vi "1DTurnMainTester.vi"() -> ()   [LabVIEW 2017]
uses:
  <vilib>/Rock Robotics/WPI/SafetyOutput/WPI_SafetyOutputConfigMenu.ctl
  <vilib>/Rock Robotics/SystemInterfaces/DIO/FPGA_DIOPWMChannel.ctl
  <vilib>/Rock Robotics/SystemInterfaces/DIO/FPGA_DIOChannel.ctl
  <extravilib>/ChannelInstances/Lossy Stream-c(dbl,dbl,dbl,dbl,dbl,dbl)/Write With Abort.vi
  <extravilib>/ChannelInstances/Lossy Stream-c(dbl,dbl,dbl,dbl,dbl,dbl)/Read With Abort.vi
  <extravilib>/ChannelInstances/Lossy Stream-c(dbl,dbl,dbl,dbl,dbl,dbl)/Endpoint.vi
  <extravilib>/ChannelInstances/Lossy Stream-c(dbl,dbl,dbl,dbl,dbl,dbl)/EndpointRead.vi
  <vilib>/Rock Robotics/WPI/RobotDrive/WPI_RobotDriveOpen4MotorWithSPARK.vi
  <vilib>/Rock Robotics/WPI/RobotDrive/WPI_RobotDriveOpen2MotorWithSPARK.vi
  <vilib>/Rock Robotics/WPI/Counter/WPI_CounterDigitalInputToDigitalSource.vi
  <extravilib>/ChannelInstances/Lossy Stream-c(dbl,dbl,dbl,dbl,dbl,dbl)/Instantiate.vi
  <extravilib>/ChannelInstances/Lossy Stream-c(dbl,dbl,dbl,dbl,dbl,dbl)/)Channel.vi
  <resource>/ChannelSupport/_ChannelSupport/WaitIfNeeded.vi
  <vilib>/Rock Robotics/WPI/ThirdParty/Sensors/navX/_Processing Loop/FRIC_navX_Internal_SPI_ProcessingLoop.vi
  <extravilib>/ChannelInstances/Lossy Stream-c(dbl,dbl,dbl,dbl,dbl,dbl).lvlib
panel:
  out "Trackwidth":dbl(graph)
  in  "AutoTurnSpeed":dbl=0.55
  in  "ThingToDo":enum16{"TestTurning", "FindTrackwidth"}(ring)
  out "Encoder Position":cluster{"Distance":dbl, "CurrentAngle":dbl}(graph)={"Distance"=0.0, "CurrentAngle"=7.280000000000058}
  in  "Gains":T1={"Gains"={"FFV"=0.0059, "FFA"=0.0019, "Vel PID"={"P"=0.01, "I"=0.0, "D"=0.0}}, "Pos PID"={"P"=0.02, "I"=0.0, "D"=0.0}, "MinVoltage"=0.0, "Effective Trackwidth"=30.0} {"Pos PID"."D" format="%.3f"; "Pos PID"."I" format="%.3f"; "Pos PID"."P" format="%.3f"}
  in  "A? or B":bool=TRUE
  in  "TargetB":dbl=500.0
  out "Voltage difference":dbl(graph)=1.0
  out "Power":dbl(graph)
  out "Done?":bool
  out "Vel":cluster{"Output":dbl, "dx/dt":dbl}(graph)
  out "Angle":cluster{"Distance":dbl, "CurrentAngle":dbl}(graph)={"Distance"=0.0, "CurrentAngle"=6.750000000000796}
  in  "TargetA":dbl
  in  "MaxVel":dbl=130.0
  in  "MaxAccel":dbl=120.0
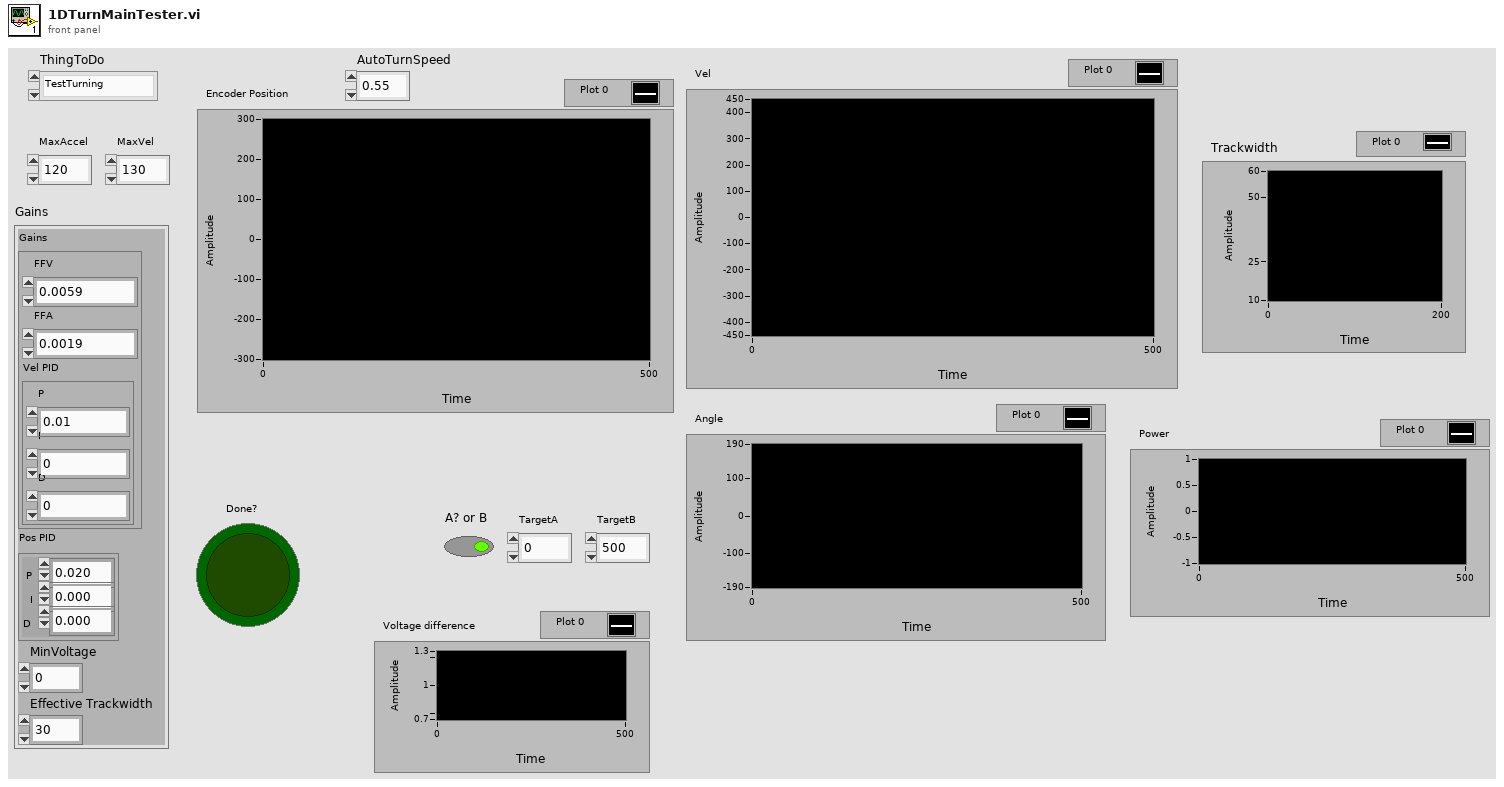
[diagram p1: front panel]
types:
  T1 = cluster{"Gains":cluster{"FFV":dbl, "FFA":dbl, "Vel PID":cluster{"P":dbl, "I":dbl, "D":dbl}}, "Pos PID":cluster{"P":dbl, "I":dbl, "D":dbl}, "MinVoltage":dbl, "Effective Trackwidth":dbl}
  T2 = typedef "FPGA_DIOChannel.ctl" = enum8{"DIO 0", "DIO 1", "DIO 2", "DIO 3", "DIO 4", "DIO 5", "DIO 6", "DIO 7", "DIO 8", "DIO 9", "DIO MXP 0", "DIO MXP 1", "DIO MXP 2", "DIO MXP 3", "DIO MXP 4", "DIO MXP 5", "DIO MXP 6", "DIO MXP 7", "DIO MXP 8", "DIO MXP 9", "DIO MXP 10", "DIO MXP 11", "DIO MXP 12", "DIO MXP 13", "DIO MXP 14", "DIO MXP 15", "SPI Port CS1", "SPI Port CS2", "SPI Port CS3", "SPI Port MISO", "SPI Port MOSI", "Invalid"}
  T3 = typedef "FPGA_DIOPWMChannel.ctl" = enum8{"PWM 0", "PWM 1", "PWM 2", "PWM 3", "PWM 4", "PWM 5", "PWM 6", "PWM 7", "PWM 8", "PWM 9", "PWM MXP 0", "PWM MXP 1", "PWM MXP 2", "PWM MXP 3", "PWM MXP 4", "PWM MXP 5", "PWM MXP 6", "PWM MXP 7", "PWM MXP 8", "PWM MXP 9", "Invalid"}
  T4 = typedef "WPI_SafetyOutputConfigMenu.ctl" = enum16{"Enable", "Disable"}
  T5 = typedef "WPI_DigitalInputDevRef.ctl" = cluster{"DevStatus":errorcluster, "DIO Channel":T2}
  T6 = typedef "FPGA_CounterEncoderSourceConvertionLVSourceType.ctl" = cluster{"DevStatus":errorcluster, "AnalogTriggerMode?":bool, "DigitalMode":cluster{"DIO Channel":T7}, "AnalogTriggerMode":cluster{"AnalogTriggerIndex":T8, "OutputType":T9}}
  T7 = typedef "FPGA_DIODigitalSourceChannel.ctl" = enum8{"DIO 0", "DIO 1", "DIO 2", "DIO 3", "DIO 4", "DIO 5", "DIO 6", "DIO 7", "DIO 8", "DIO 9", "DIO MXP 0", "DIO MXP 1", "DIO MXP 2", "DIO MXP 3", "DIO MXP 4", "DIO MXP 5", "DIO MXP 6", "DIO MXP 7", "DIO MXP 8", "DIO MXP 9", "DIO MXP 10", "DIO MXP 11", "DIO MXP 12", "DIO MXP 13", "DIO MXP 14", "DIO MXP 15", "Disabled"}
  T8 = typedef "FPGA_AnalogTriggerIndex.ctl" = enum8{"Trig 0", "Trig 1", "Trig 2", "Trig 3", "Trig 4", "Trig 5", "Trig 6", "Trig 7", "Invalid"}
  T9 = typedef "FPGA_AnalogTriggerOutType.ctl" = enum16{"InWindow", "TriggerState", "Rising", "Falling"}
  T10 = typedef "WPI_EncoderDevRef.ctl" = cluster{"DevStatus":errorcluster, "EncoderIndex":T11, "CounterIndex":T12, "DistancePerCount":dbl, "Decoding Type":T13}
  T11 = typedef "FPGA_EncoderIdx.ctl" = enum8{"Enc 0", "Enc 1", "Enc 2", "Enc 3", "Enc 4", "Enc 5", "Enc 6", "Enc 7", "Invalid"}
  T12 = typedef "FPGA_CounterCtrSystemIndex.ctl" = enum8{"Ctr 0", "Ctr 1", "Ctr 2", "Ctr 3", "Ctr 4", "Ctr 5", "Ctr 6", "Ctr 7", "Invalid"}
  T13 = typedef "WPI_EncoderType.ctl" = enum16{"1x", "2x", "4x"}
  T14 = typedef "WPI_RobotDriveDevRef.ctl" = cluster{"DevStatus":errorcluster, "Motors[]":T15[], "Square Inputs":bool, "Max Output":dbl}
  T15 = typedef "WPI_MotorControlDeviceRef.ctl" = cluster{"DeviceStatus":errorcluster, "Type":T16, "PWM":cluster{"PWM Channel":T3, "DeadBand":T17}, "CAN":cluster{"Device Number":u8, "SetOutput VI Ref":variant, "GetOutput VI Ref":variant, "Enable VI Ref":variant, "Disable VI Ref":variant, "Data":variant}, "Invert":bool, "DIO PWM":cluster{"PWM \"Enable\" Channel":T3, "DIOChannel":T2, "PWM Rate":dbl}}
  T16 = typedef "WPI_MotorControlType.ctl" = enum16{"PWM", "CAN", "DIO PWM"}
  T17 = typedef "WPI_PWMDeadband.ctl" = cluster{"Name":string, "maxPositivePwm":i32, "minPositivePwm":i32, "centerPwm":i32, "maxNegativePwm":i32, "minNegativePwm":i32, "angularRange":u16}
  T18 = cluster{"Yaw":dbl, "Roll":dbl, "Pitch":dbl, "Heading":dbl, "Fused Heading":dbl}
  T19 = cluster{dbl, "dx/dt":dbl, "Distance":dbl, "dx/dt":dbl, "Distance":dbl, "dx/dt":dbl}
  T20 = typedef "Lossy Stream-c(dbl,dbl,dbl,dbl,dbl,dbl).lvlib/)Channel.ctl" = refnum<queue>
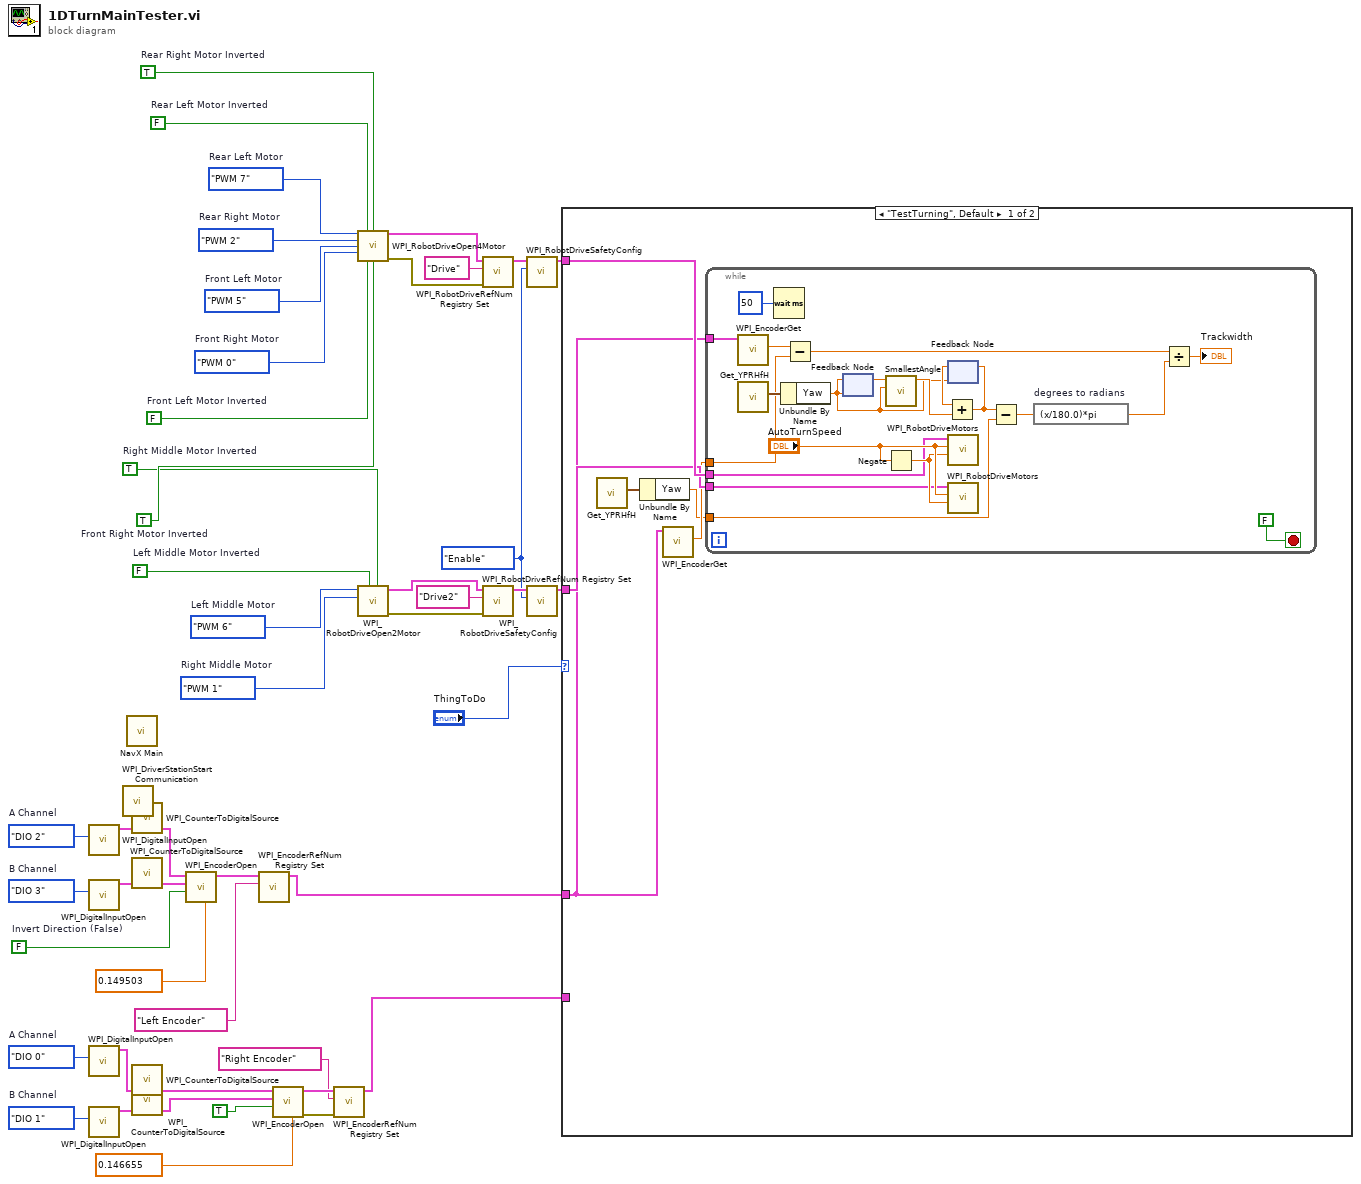
[diagram p0: block diagram]
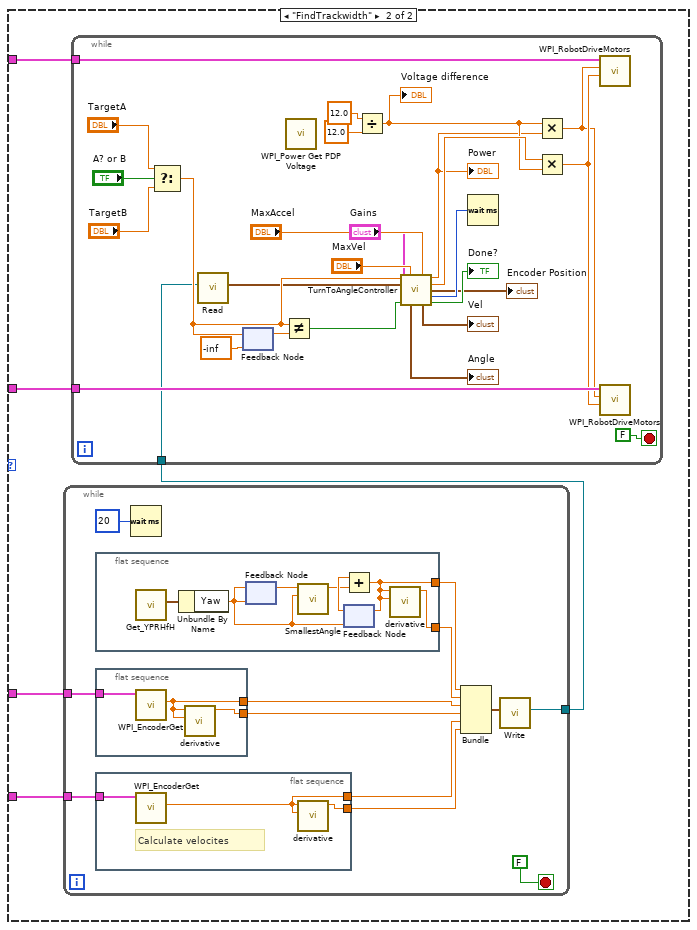
[diagram p2: hidden frame]
diagram:
  w7 = FPGA_DIOChannel."DIO 1"  # B Channel
  w10 = FPGA_DIOChannel."DIO 0"  # A Channel
  w23 = FALSE  # Invert Direction (False)
  w16 = FPGA_DIOChannel."DIO 3"  # B Channel
  w17 = FPGA_DIOChannel."DIO 2"  # A Channel
  w32 = TRUE  # Right Middle Motor Inverted
  w33 = FALSE  # Left Middle Motor Inverted
  w27 = FPGA_DIOPWMChannel."PWM 1"  # Right Middle Motor
  w36 = FPGA_DIOPWMChannel."PWM 6"  # Left Middle Motor
  w37 = TRUE  # Front Right Motor Inverted
  w38 = FALSE  # Front Left Motor Inverted
  w39 = TRUE  # Rear Right Motor Inverted
  w40 = FALSE  # Rear Left Motor Inverted
  w41 = FPGA_DIOPWMChannel."PWM 0"  # Front Right Motor
  w42 = FPGA_DIOPWMChannel."PWM 5"  # Front Left Motor
  w43 = FPGA_DIOPWMChannel."PWM 2"  # Rear Right Motor
  w44 = FPGA_DIOPWMChannel."PWM 7"  # Rear Left Motor
  w28 = WPI_SafetyOutputConfigMenu."Enable" ("mode")
  n1 = call <vilib>:"WPI_DigitalInputOpen.vi"("DIO Channel"=w17) -> ("DigitalInputDevRef"=w20:T5)  [unwired: 1 in, 9 out]
  n2 = call <vilib>:"WPI_DigitalInputOpen.vi"("DIO Channel"=w16) -> ("DigitalInputDevRef"=w19:T5)  [unwired: 1 in, 9 out]
  n3 = call <vilib>:"WPI_DigitalInputOpen.vi"("DIO Channel"=w10) -> ("DigitalInputDevRef"=w11:T5)  [unwired: 1 in, 9 out]
  n4 = call <vilib>:"WPI_DigitalInputOpen.vi"("DIO Channel"=w7) -> ("DigitalInputDevRef"=w8:T5)  [unwired: 1 in, 9 out]
  n5 = call <vilib>:"WPI_DriverStationStart Communication.vi"() -> ()  [unwired: 12 in]
  n6 = call-poly <vilib>:"NavX Main.vi"() -> ()  [unwired: 12 in]
  n7 = call-poly <vilib>:"WPI_CounterToDigitalSource.vi"("DigitalInputDevRef"=w20) -> ("Digital Source"=w21:T6)  [unwired: 6 out]
  n8 = call-poly <vilib>:"WPI_CounterToDigitalSource.vi"("DigitalInputDevRef"=w19) -> ("Digital Source"=w18:T6)  [unwired: 6 out]
  n9 = call-poly <vilib>:"WPI_CounterToDigitalSource.vi"("DigitalInputDevRef"=w11) -> ("Digital Source"=w12:T6)  [unwired: 6 out]
  n10 = call-poly <vilib>:"WPI_CounterToDigitalSource.vi"("DigitalInputDevRef"=w8) -> ("Digital Source"=w9:T6)  [unwired: 6 out]
  n11 = call <vilib>:"WPI_EncoderOpen.vi"("DistancePerCount"=0.149503, "Invert Direction (False)"=w23, "BSource"=w18, "ASource"=w21) -> ("EncoderDevRef"=w22:T10)  [unwired: 4 in, 3 out]
  n12 = call <vilib>:"WPI_EncoderRefNum Registry Set.vi"("refnum name"="Left Encoder", "EncoderDevRef"=w22) -> ("EncoderDevRef"=w3:T10)  [unwired: 8 in, 1 out]
  n13 = call <vilib>:"WPI_EncoderOpen.vi"("DistancePerCount"=0.146655, "Invert Direction (False)"=TRUE, "BSource"=w9, "ASource"=w12) -> ("error out"=w14:errorcluster, "EncoderDevRef"=w13:T10)  [unwired: 4 in, 2 out]
  n14 = call <vilib>:"WPI_EncoderRefNum Registry Set.vi"("error in (no error)"=w14, "refnum name"="Right Encoder", "EncoderDevRef"=w13) -> ("EncoderDevRef"=w2:T10)  [unwired: 7 in, 1 out]
  n15 = call-poly <vilib>:"WPI_RobotDriveOpen4Motor.vi"("Rear Left Motor"=w44, "Rear Left Motor Inverted"=w40, "Rear Right Motor Inverted"=w39, "Rear Right Motor"=w43, "Front Left Motor"=w42, "Front Right Motor"=w41, "Front Left Motor Inverted"=w38, "Front Right Motor Inverted"=w37) -> ("RobotDriveDevRef"=w47:T14, "error out"=w45:errorcluster)  [unwired: 6 in]
  n16 = call-poly <vilib>:"WPI_RobotDriveOpen2Motor.vi"("Right Motor Inverted"=w32, "Left Motor Inverted"=w33, "Right Motor"=w27, "Left Motor"=w36) -> ("error out"=w31:errorcluster, "RobotDriveDevRef"=w35:T14)  [unwired: 6 in]
  n17 = call <vilib>:"WPI_RobotDriveRefNum Registry Set.vi"("error in (no error)"=w45, "refnum name"="Drive", "RobotDriveDevRef"=w47) -> ("RobotDriveDevRef"=w30:T14)  [unwired: 1 in, 7 out]
  n18 = call <vilib>:"WPI_RobotDriveRefNum Registry Set.vi"("error in (no error)"=w31, "refnum name"="Drive2", "RobotDriveDevRef"=w35) -> ("RobotDriveDevRef"=w29:T14)  [unwired: 7 in, 1 out]
  n19 = call <vilib>:"WPI_RobotDriveSafetyConfig.vi"("mode"=w28, "RobotDriveDevRef"=w30) -> ("RobotDriveDevRef"=w25:T14)  [unwired: 8 in, 1 out]
  n20 = call <vilib>:"WPI_RobotDriveSafetyConfig.vi"("mode"=w28, "RobotDriveDevRef"=w29) -> ("RobotDriveDevRef"=w26:T14)  [unwired: 8 in, 1 out]
  n21 = case shown="\"TestTurning\", Default" "ThingToDo" {
    tunnel: w26 -> [w52 w78]
    tunnel: w25 -> [w53 w77]
    tunnel: w3 -> [w51 w76]
    tunnel: w2 -> [_ w75]
    frame "TestTurning", Default {
      n22 = call <vilib>:"Get_YPRHfH.vi"() -> ("YRPHfH"=w49:T18)  [unwired: 11 in]
      n23 = Unbundle By Name(w49) -> ("Yaw"=w48:dbl)
      n24 = call <vilib>:"WPI_EncoderGet.vi"("EncoderDevRef"=w51) -> ("Distance"=w50:dbl)  [unwired: 5 in, 5 out]
      n25 = while {
        tunnel: w53 -> [w69]
        tunnel: w52 -> [w68]
        tunnel: w51 -> [w62]
        tunnel: w50 -> [w60]
        tunnel: w48 -> [w58]
        stop <- FALSE stop-if-true
        n26 = call <vilib>:"WPI_EncoderGet.vi"("EncoderDevRef"=w62) -> ("Distance"=w61:dbl)  [unwired: 5 in, 5 out]
        n27 = call <vilib>:"Get_YPRHfH.vi"() -> ("YRPHfH"=w67:T18)  [unwired: 11 in]
        n28 = Wait (ms)(milliseconds to wait=u32 50) -> ()  [unwired: 1 out]
        n29 = Unbundle By Name(w67) -> ("Yaw"=w63:dbl)
        n30 = Subtract(x=w61, y=w60) -> (x-y=w56:dbl)
        n31 = feedback #1(w63) -> (w64:dbl)
        n32 = feedback-in #1(w63) -> ()
        n33 = call "SmallestAngle.vi"("Angle B"=w63, "Angle A"=w64) -> ("Smallest A to B"=w65:dbl)  [unwired: 9 in]
        n34 = Negate(x="AutoTurnSpeed") -> (-x=w72:dbl)
        n35 = feedback #2(w63) -> (w66:dbl)
        n36 = Add(x=w66, y=w65) -> (x+y=w59:dbl)
        n37 = feedback-in #2(w59) -> ()
        n38 = call <vilib>:"WPI_RobotDriveMotors.vi"("RightSpeed"=w72, "LeftSpeed"="AutoTurnSpeed", "RobotDriveDevRef"=w69) -> ()  [unwired: 1 in, 8 out]
        n39 = call <vilib>:"WPI_RobotDriveMotors.vi"("RightSpeed"=w72, "LeftSpeed"="AutoTurnSpeed", "RobotDriveDevRef"=w68) -> ()  [unwired: 1 in, 8 out]
        n40 = Subtract(x=w59, y=w58) -> (x-y=w57:dbl)
        n41 = expression code="(x/180.0)*pi" "degrees to radians"(w57) -> (w55:dbl)
        n42 = Divide(x=w56, y=w55) -> (x/y=→"Trackwidth":dbl)
      }
    }
    frame "FindTrackwidth" {
      n43 = while {
        tunnel: w76 -> [w86]
        tunnel: w75 -> [w85]
        tunnel: [w79] -> w74
        stop <- FALSE stop-if-true
        n44 = flat-sequence {
          tunnel: [w102] -> w87
          tunnel: [w98] -> w88
          frame #0 {
            n45 = call <vilib>:"Get_YPRHfH.vi"() -> ("YRPHfH"=w103:T18)  [unwired: 11 in]
            n46 = Unbundle By Name(w103) -> ("Yaw"=w97:dbl)
            n47 = feedback #3(w97) -> (w99:dbl)
            n48 = feedback-in #3(w97) -> ()
            n49 = call "SmallestAngle.vi"("Angle B"=w97, "Angle A"=w99) -> ("Smallest A to B"=w100:dbl)  [unwired: 9 in]
            n50 = feedback #4(w97) -> (w101:dbl)
            n51 = Add(x=w101, y=w100) -> (x+y=w98:dbl)
            n52 = feedback-in #4(w98) -> ()
            n53 = call "derivative.vi"("Starting value"=w98, "x"=w98) -> ("dx/dt"=w102:dbl)  [unwired: 9 in]
          }
        }
        n54 = flat-sequence {
          tunnel: [w93] -> w83
          tunnel: [w92] -> w84
          tunnel: w86 -> [w91]
          frame #0 {
            n55 = call <vilib>:"WPI_EncoderGet.vi"("EncoderDevRef"=w91) -> ("Distance"=w92:dbl)  [unwired: 5 in, 5 out]
            n56 = call "derivative.vi"("Starting value"=w92, "x"=w92) -> ("dx/dt"=w93:dbl)  [unwired: 9 in]
          }
        }
        n57 = flat-sequence {
          tunnel: [w95] -> w81
          tunnel: [w94] -> w82
          tunnel: w85 -> [w96]
          frame #0 {
            # "Calculate velocites"
            n58 = call <vilib>:"WPI_EncoderGet.vi"("EncoderDevRef"=w96) -> ("Distance"=w94:dbl)  [unwired: 5 in, 5 out]
            n59 = call "derivative.vi"("Starting value"=w94, "x"=w94) -> ("dx/dt"=w95:dbl)  [unwired: 9 in]
          }
        }
        n60 = Wait (ms)(milliseconds to wait=u32 20) -> ()  [unwired: 1 out]
        n61 = Bundle(w88, "dx/dt"=w87, "Distance"=w84, "dx/dt"=w83, "Distance"=w82, "dx/dt"=w81) -> (w80:T19)  [unwired: 1 in]
        n62 = call <extravilib>:"Write.vi"("element"=w80) -> ("channel"=w79:T20)  [unwired: 8 in, 2 out]
      }
      n63 = while {
        tunnel: w78 -> [w121]
        tunnel: w77 -> [w120]
        tunnel: w74 -> [w108]
        stop <- FALSE stop-if-true
        n64 = Select(t="TargetA", s="A? or B", f="TargetB") -> (s? t:f=w109:dbl)
        n65 = call <extravilib>:"Read.vi"("channel"=w108) -> ("element"=w107:T19)  [unwired: 5 in, 5 out]
        n66 = feedback-in #5(w109) -> ()
        n67 = feedback #5(-inf ("TargetAngle")) -> (w123:dbl)
        n68 = Not Equal?(x=w109, y=w123) -> (x != y?=w122:bool)
        n69 = call <vilib>:"WPI_Power Get PDP Voltage.vi"() -> ()  [unwired: 14 in, 2 out]
        n70 = Divide(x=12.0, y=12.0) -> (x/y=w115:dbl)
        "Voltage difference" <- w115
        n71 = call "TurnToAngleController.vi"("TargetAngle"=w109, "MaxVel"="MaxVel", "MaxAccel"="MaxAccel", "Robot"=w107, "Gains"="Gains", "Reset"=w122) -> ("LeftPower"=w105:dbl, "RightPower"=w117:dbl, "Encoder Position"=→"Encoder Position":cluster{"Distance":dbl, "CurrentAngle":dbl}, "Delay"=w129:u32, "Angle"=→"Angle":cluster{"Distance":dbl, "CurrentAngle":dbl}, "VelGraph"=→"Vel":cluster{"Output":dbl, "dx/dt":dbl}, "Done"=→"Done?":bool)  [unwired: 3 in]
        "Power" <- w105
        n72 = Wait (ms)(milliseconds to wait=w129) -> ()  [unwired: 1 out]
        n73 = Multiply(x=w115, y=w105) -> (x*y=w114:dbl)
        n74 = Multiply(x=w117, y=w115) -> (x*y=w116:dbl)
        n75 = call <vilib>:"WPI_RobotDriveMotors.vi"("RightSpeed"=w116, "LeftSpeed"=w114, "RobotDriveDevRef"=w120) -> ()  [unwired: 1 in, 8 out]
        n76 = call <vilib>:"WPI_RobotDriveMotors.vi"("RightSpeed"=w116, "LeftSpeed"=w114, "RobotDriveDevRef"=w121) -> ()  [unwired: 1 in, 8 out]
      }
    }
  }
